vi "Add.vi"(8 "error in (no error)":errorcluster caption="错误输入（无错误）", 11 "ê ÁÐÝ”Èë":refnum<queue>) -> (0 "error out":errorcluster caption="错误输出")   [LabVIEW 2012]
uses:
  SupportVi/SystemState.ctl
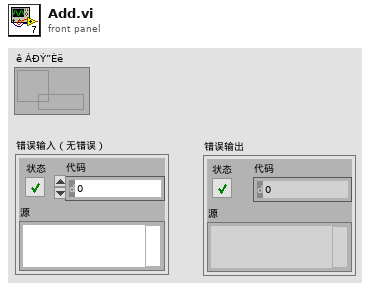
[diagram p1: front panel]
types:
  T1 = typedef "SystemState.ctl" = enum16{"Quit", "Error", "Stopping", "Starting", "Init", "Scan", "Menu", "ReadConf", "Idle"}
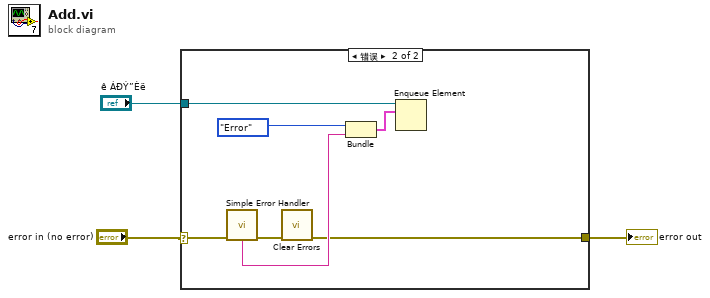
[diagram p0: block diagram]
diagram:
  n1 = case shown="错误" "error in (no error)" {
    selector: "error in (no error)" -> [w4 w11]
    tunnel: "ê ÁÐÝ”Èë" -> [_ w9]
    tunnel: [w4 w5] -> w1
    frame No Error {
    }
    frame Error {
      n2 = call <vilib>:"Simple Error Handler.vi"("error in (no error)"=w11) -> ("error out"=w10:errorcluster, "message"=w6:string)  [unwired: 4 in, 3 out]
      n3 = call <vilib>:"Clear Errors.vi"("error in (no error)"=w10) -> ("error out"=w5:errorcluster)  [unwired: 6 in]
      n4 = Bundle("î‘B"=SystemState."Error", "message"=w6) -> (w8:cluster{" î‘B":T1, "message":string})  [unwired: 1 in]
      n5 = Enqueue Element(queue=w9, element=w8) -> ()  [unwired: 2 in, 3 out]
    }
  }
  "error out" <- w1
